vi "Dashboard Main.vi"() -> ()   [LabVIEW 2016]
uses:
  <vilib>/event_ctls.llb/eventvkey.ctl
  <vilib>/Rock Robotics/WPI/Dashboard/WPI_DashboardLogging Global.vi
  <vilib>/Utility/config.llb/Write Key (String).vi
  <vilib>/Utility/config.llb/Write Key (I32).vi
  <vilib>/Utility/config.llb/NI_LVConfig.lvlib
panel:
  out "Camera IP":string
  in  "TCP":refnum<k5>
  in  "Rec Mode":enum32{"Stop", "Record", "Playback"}(radio)
  in  "Vision":u16(ring) items=["Camera Off", "USB Camera SW", "USB Camera HW", "IP Camera"]
  out "Image Message":string="Timeout in Camera Communications"
  in  "Dashboard Tab":T1(tab)
  out "Feeder":bool
  out "GearPickupDown":bool caption="Gear Down"
  out "TargetLocked":bool caption="Locked"
  out "AutoTarget":bool caption="Target\nTarget"
  out "GearPickupMotor":bool caption="Gear Pickup"
  out "BallPickupMotor":bool caption="Ball Pickup"
  out "ShooterMotor":bool caption="Shooter"
  out "PTO":bool
  out "Neutral":bool
  out "High":bool caption="High Gear"
  out "Low":bool caption="Low Gear"
  in  "CompressorEnabled":bool caption="Compressor"
  out "Compressor":bool
  in  "AutoProgramSelect":u16(ring) items=["0 - No Auto Program", "1 - Drive to Line and Stop", "2 - Place Gear Center", "3 - Place Gear Start Left", "4 - Place Gear Start Right", "5 - Place Gear Vision Start Left", "6 - Place Gear Vision Start Right", "7 - Test Backwards Driving"]
  out "Low Battery":bool
  out "FMS":bool
  out "Teleop Mode":bool
  out "Auto Mode":bool
  out "Disabled":bool
  in  "Program":string
  in  "Camera Settings Old":T2={"Frame Rate"=30, "Compression"=30, "Size"=1, "Boolean"=FALSE} {"Frame Rate" scale=1.0..30.0; "Size" items=["640x480", "320x240", "160x120"]}
  out "Mode":T3(ring)=enum."Auto Disabled"
  in  "DB Camera Config":bool
  out "fps":dbl format="%#.1g"
  out "Mbps":dbl format="%#.1g"
  out "Mbps 2":bool
  in  "PIDEnabled":bool caption="PID Enabled"
  in  "LCD_Line_10":string caption="DB/String 0"
  in  "LCD_Line_9":string caption="DB/String 0"
  in  "LCD_Line_8":string caption="DB/String 0"
  in  "LCD_Line_7":string caption="DB/String 0"
  in  "LCD_Line_6":string caption="DB/String 0"
  in  "LCD_Line_5":string caption="DB/String 0"
  in  "LCD_Line_4":string caption="DB/String 0"
  in  "LCD_Line_3":string caption="DB/String 0"
  in  "LCD_Line_2":string caption="DB/String 0"
  in  "LCD_Line_1":string caption="DB/String 0"
  in  "PValue":dbl caption="P"
  in  "IValue":dbl caption="I"
  in  "DValue":dbl caption="D"
  in  "LowSetting":dbl caption="Low"
  in  "HighSetting":dbl caption="High"
  in  "DB/String 9":string
  in  "DB/String 8":string
  in  "DB/String 7":string
  in  "DB/String 6":string
  in  "DB/String 5":string
  in  "DB/String 4":string
  in  "DB/String 3":string
  in  "DB/String 2":string
  in  "DB/String 1":string
  in  "DB/String 0":string
  in  "DB/Slider 0":dbl(slide) scale=0.0..5.0
  in  "DB/Slider 1":dbl(slide) scale=0.0..5.0
  in  "DB/Slider 2":dbl(slide) scale=0.0..5.0
  in  "DB/Slider 3":dbl(slide) scale=0.0..5.0
  out "DB/LED 3":bool
  out "DB/LED 2":bool
  out "DB/LED 1":bool
  out "DB/LED 0":bool
  in  "DB/Button 3":bool
  in  "DB/Button 2":bool
  in  "DB/Button 1":bool
  in  "DB/Button 0":bool caption="New Name"
  in  "Test Slider":dbl(slide) scale=0.0..100.0 scale format="%#_3g"
  in  "On/Off":bool caption="Solenoid"
  in  "Test Name":u16(ring) items=["Select the test to run...", "Example Test", "-------------------------------", "List of tests is built in robot code.", "Replace with your own automated tests."]
  in  "Test Tree":string(tree)
  in  "Motor":cluster{"Value":dbl, "Enable":bool} {"Value" scale=-1.0..1.0 scale format="%#_3g"}
  out "Progress":T4 {"Test Progress" scale=0.0..100.0}
  in  "Rev/Fwd":cluster{"Forward":bool, "Reverse":bool}
  in  "Test Ring":u16(ring) items=["Monochrome", "Color"]
  in  "Listbox":i32(listbox)
  out "Tree":string(tree)
  out "Camera Image":T5(plugin-control)
  out "Boolean":bool
  # "Program:"
  # "Dashboard: 2017-04"
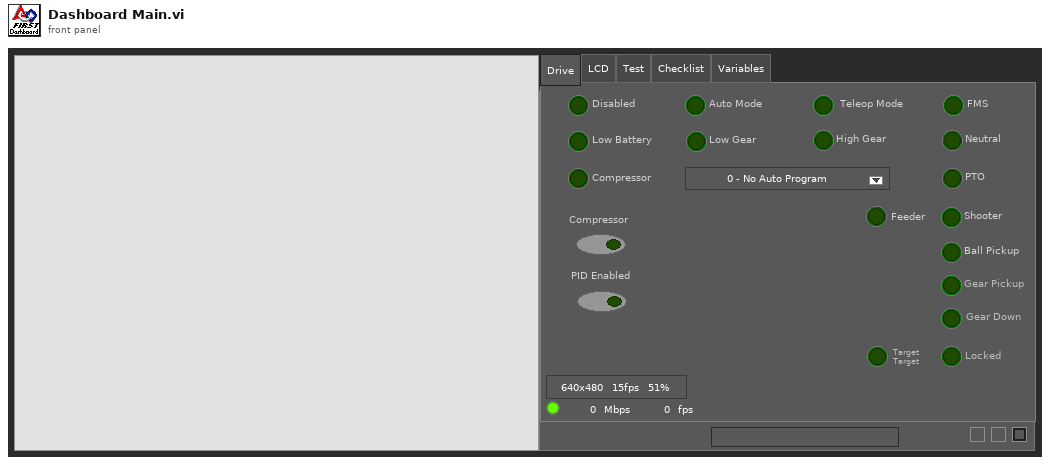
[diagram p1: front panel]
types:
  T1 = enum32{"Drive", "LCD", "Basic", "Test", "Checklist", "Variables"}
  T2 = cluster{"Frame Rate":i32, "Compression":i32, "Size":u16, "Boolean":bool}
  T3 = enum8{"Tele-Op Disabled", "Tele-Op Enabled", "Auto Disabled", "Auto Enabled", "Test Disabled", "Test Enabled", "Disconnected", "No Code", "E-Stop"}
  T4 = cluster{"Test Progress":u8, "Test Progress Text":string}
  T5 = typedef "IMAQ Image.ctl" = refnum<image>
  T6 = enum32{"Drive", "Basic", "Custom", "Test", "Checklist", "Variables"}
  T7 = typedef "Image Type" = u32
  T8 = cluster{"Camera Image":refnum<vi>, "Dashboard Tab":refnum<vi>, "Boolean":refnum<vi>, "Vision":refnum<vi>, "Rec Mode":refnum<vi>, "Test Slider":refnum<vi>, "On/Off ":refnum<vi>, "Test Ring":refnum<vi>, "Rev/Fwd":refnum<vi>, "Test Name":refnum<vi>, "Motor":refnum<vi>, "Progress":refnum<vi>, "CheckList":refnum<vi>, "Tree":refnum<vi>, "Test Tree":refnum<vi>}
  T9 = cluster{"Error Strings":string, "Disable Counts":cluster{u16, u16}, "Rail Faults":cluster{u16, u16, u16}, "Robot IP":string, "DB Mode":u8, "Event Info":cluster{"Name":string, "Type":u8, "Number":u16, "Replay":u8}}
  T10 = cluster{"Storage":cluster{"Disk Free":u64, "RAM Block":u32, "RAM free":u32}, "CPU Utilization":cluster{"CPU % ISR":sgl, "CPU % Time Crit":sgl, "CPU % Timed Str":sgl, "CPU % High":sgl, "CPU % Above":sgl, "CPU % Normal":sgl, "CPU % Low":sgl}, "CAN":cluster{"% Bus Utilization":sgl, "Bus Off Cnt":u32, "TX_FIFO Full Cnt":u32, "Receive Error Cnt":u8, "Transmit Error Cnt":u8}, "HID":cluster{"HID Outputs":u32, "Rumble Low":u16, "Rumble High":u16}[]}
  T11 = cluster{"Status bits":cluster{"Test Mode":bool, "Autonomous":bool, "Enabled":bool, "Code Start":bool, "Brownout":bool, "Reserved 2":bool, "Reserved 3":bool, "E-Stop":bool}, "Code Trace":cluster{"Disabled":bool, "TeleOp":bool, "Auto":bool, "Test":bool}, "Controller Type":enum16{"unknown", "cRIO", "roboRio"}, "Code?":enum16{"unknown", "noCode", "code"}, "Battery V":dbl}
  T12 = cluster{"Control Bits":cluster{"TestMode":bool, "Autonomous":bool, "Enabled":bool, "FMS Present":bool, bool, bool, bool, "E-Stop":bool}, "Team Station ":u8, "Countdown":sgl, "Joystick Values":cluster{"Axes":dbl[], "Buttons":bool[], "POVs":i16[]}[]}
  T13 = cluster{"value":i32, "value":i32, "index":i32, "Boolean":bool}
  T14 = typedef "NI_LVConfig.lvlib/Config Data RefNum.ctl" = refnum<k1>
  T15 = cluster{"Operation":enum16{"Update", "Clear"}, "Color Box":u32}[]
  T16 = typedef "eventvkey.ctl" = enum16{"ASCII", "Enter", "Return", "Shift", "Ctrl", "Alt", "Cmd", "Opt", "Caps", "NumLock", "Clear", "Break", "Up", "Down", "Left", "Right", "Insert", "Delete", "Home", "End", "PageUp", "PageDown", "Escape", "Help", "Pause", "ScrollLock", "F1", "F2", "F3", "F4", "F5", "F6", "F7", "F8", "F9", "F10", "F11", "F12", "F13", "F14", "F15", "F16", "F17", "F18", "F19", "F20", "F21", "F22", "F23", "F24", "Play", "VolumeUp", "VolumeDown", "Mute", "Two Byte Char"}
  T17 = cluster{"Image Size":bool, "Image Type":bool, "Pixel Value":bool, "ROI Information":bool, "Zoom Factor":bool}
  T18 = enum8{"Enabled", "Disabled", "Disabled and Grayed Out"}
  T19 = cluster{"Operation":enum16{"Update", "Clear"}, "Color Box":u32}
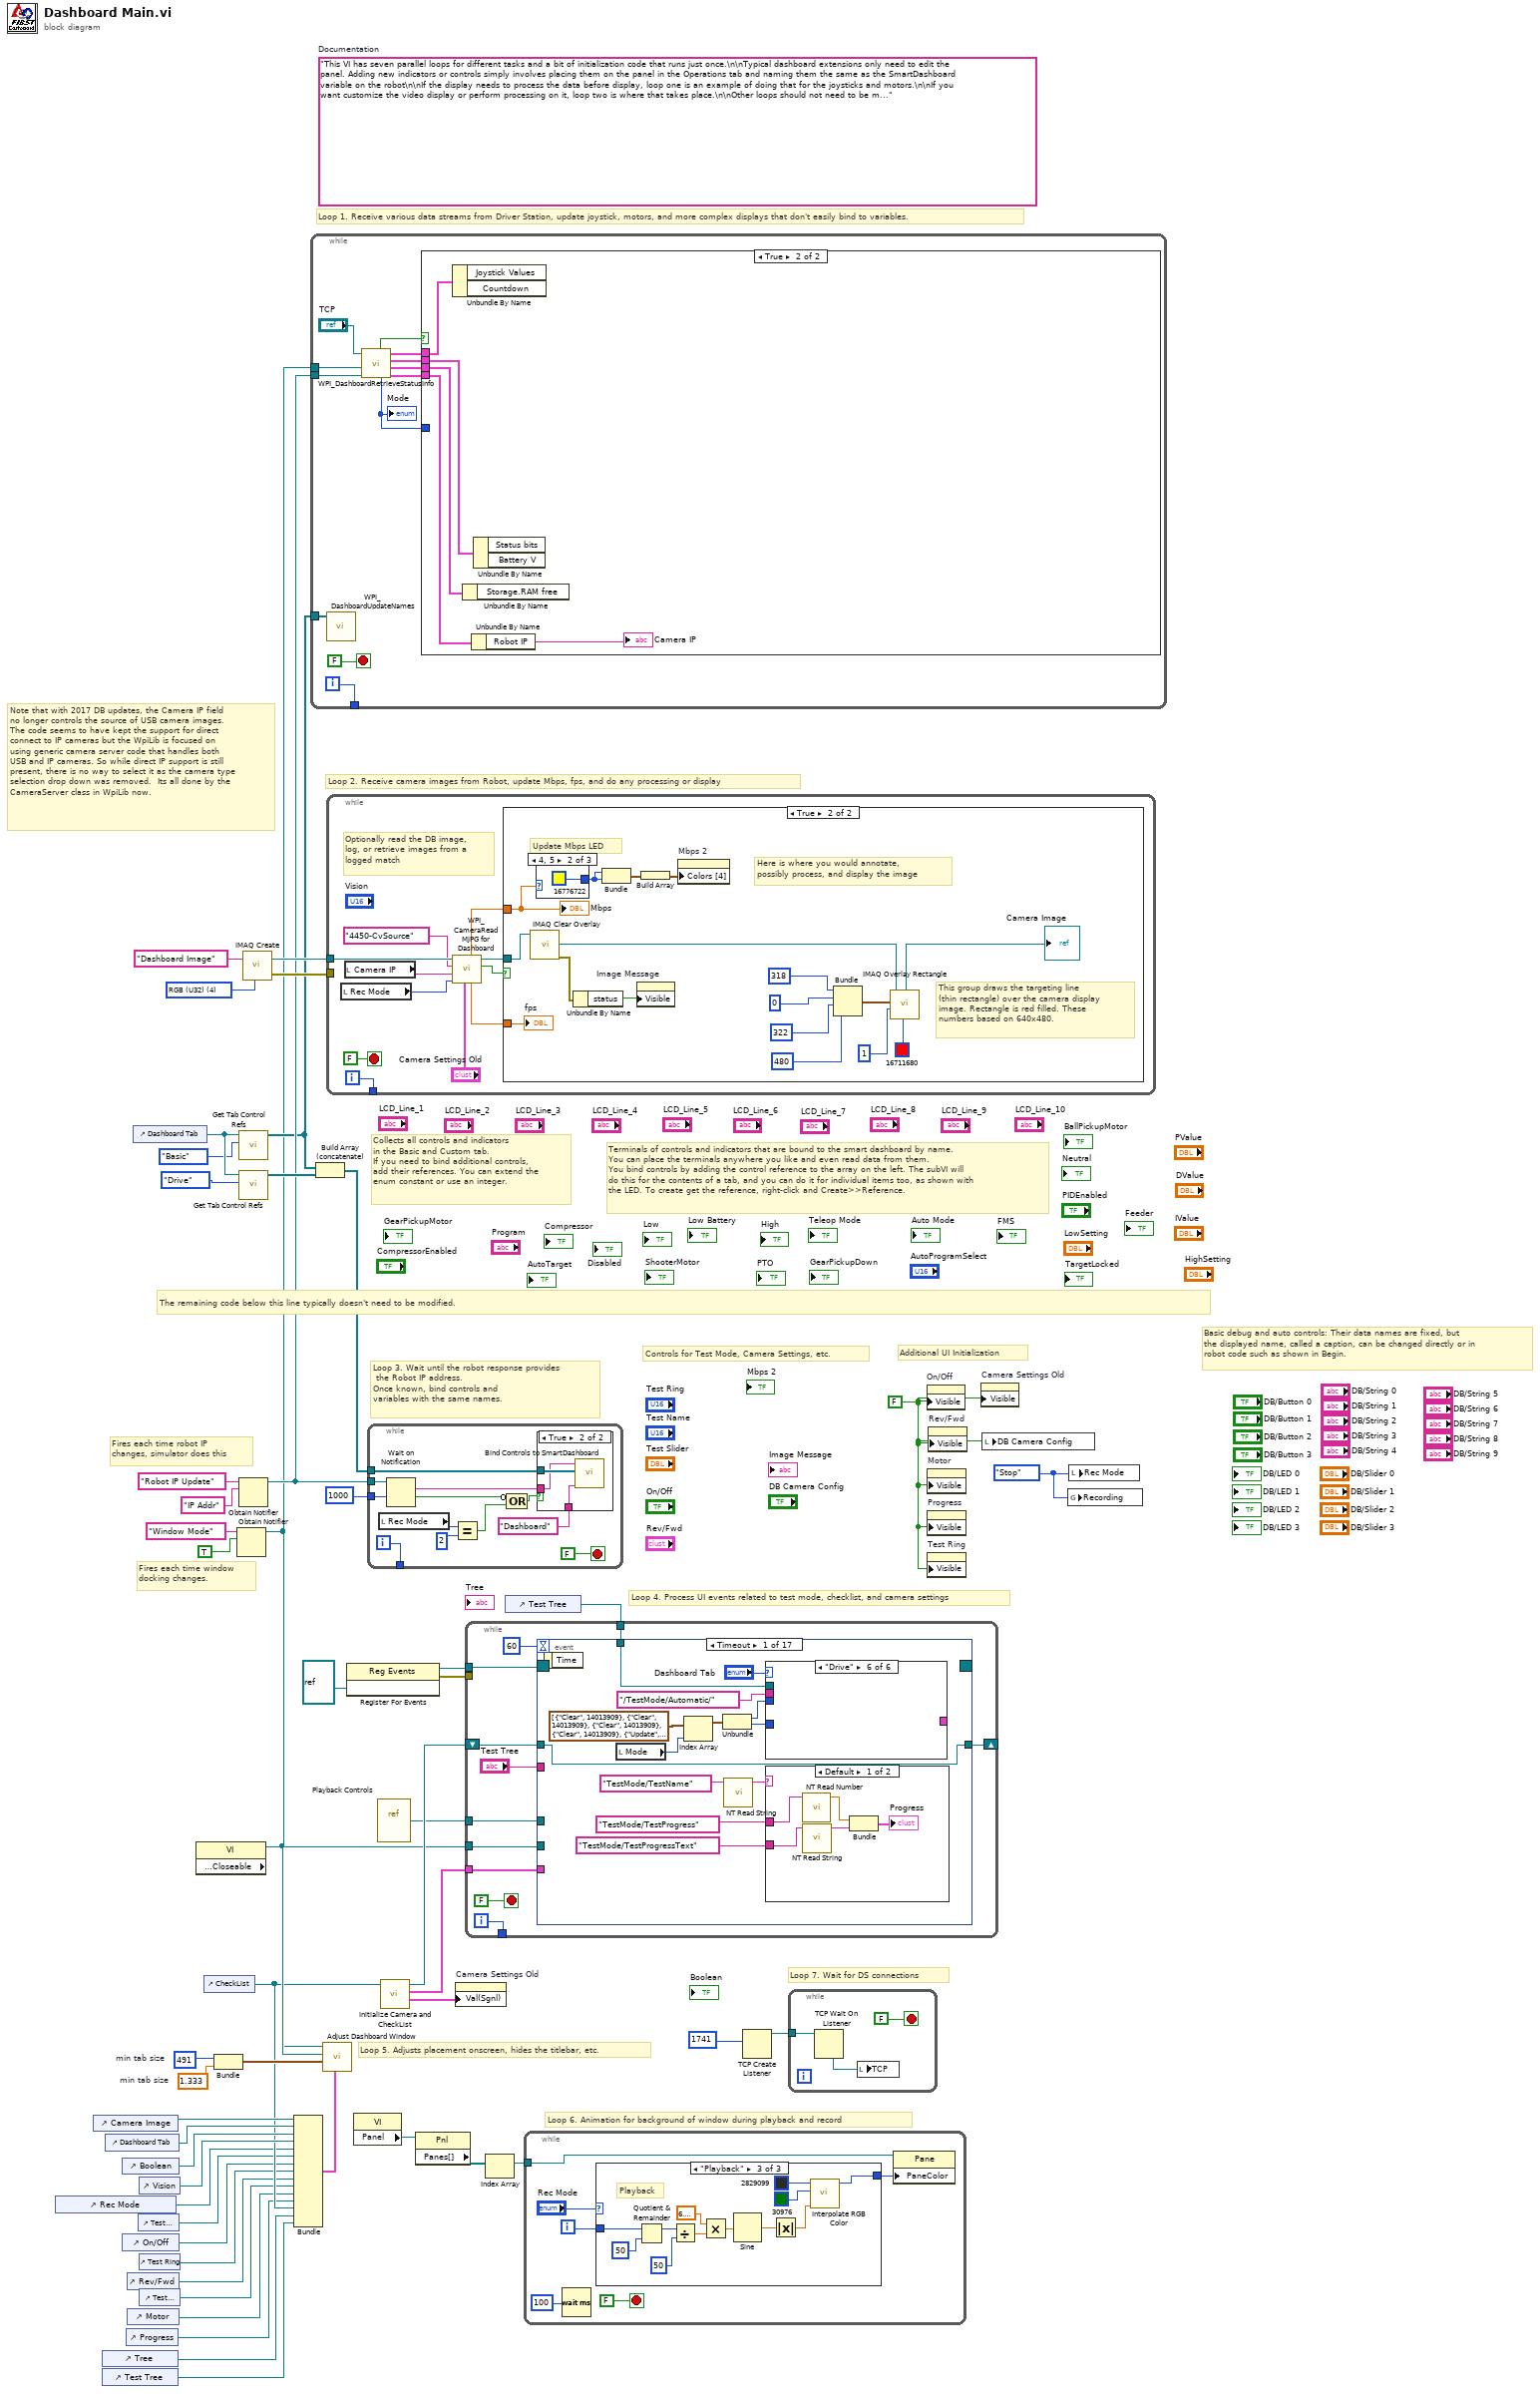
[diagram p0: block diagram]
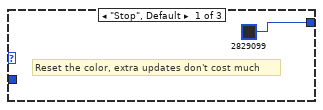
[diagram p3: hidden frame]
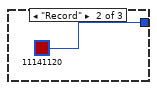
[diagram p4: hidden frame]
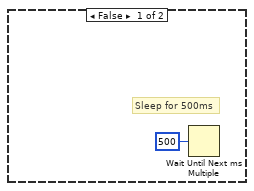
[diagram p6: hidden frame]
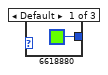
[diagram p7: hidden frame]
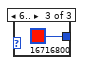
[diagram p8: hidden frame]
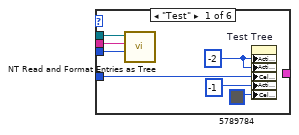
[diagram p9: hidden frame]
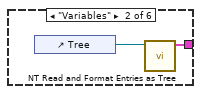
[diagram p10: hidden frame]
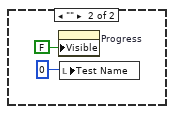
[diagram p14: hidden frame]
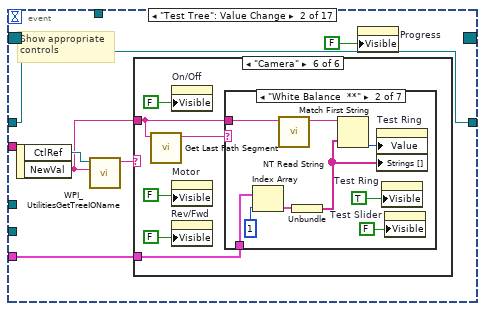
[diagram p15: hidden frame]
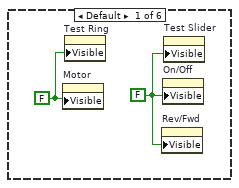
[diagram p16: hidden frame]
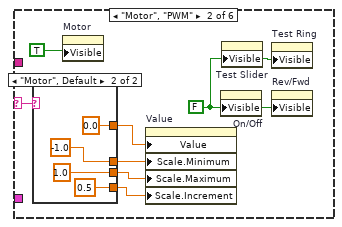
[diagram p17: hidden frame]
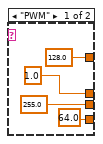
[diagram p18: hidden frame]
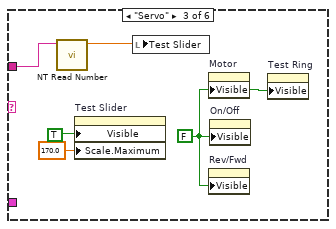
[diagram p19: hidden frame]
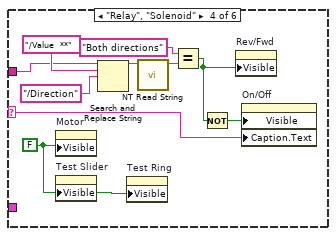
[diagram p20: hidden frame]
diagram:
  w24 = 491  # min tab size
  w23 = 1.333  # min tab size
  w32 = enum32{"Stop", "Record", "Playback"}."Stop" ("Rec Mode")
  w6 = FALSE ("Visible")
  (unwired) "This VI has seven parallel loops for different tasks and a bit of initialization code that runs just once.\n\nTypical dashboard extensions only need to edit the panel. Adding new indicators or controls simply involves placing them on the panel in the Operations tab and naming them the same as the SmartDashboard variable on the robot\n\nIf the display needs to process the data before display, loop one is an example of doing that for the joysticks and motors.\n\nIf you want customize the video display or perform processing on it, loop two is where that takes place.\n\nOther loops should not need to be modified. They are pretty standard, and document the task they perform."  # Documentation
  w52 = T7 4 items=["Grayscale (U8)", "Grayscale (I16)", "Grayscale (SGL)", "Complex (CSG)", "RGB (U32)", "HSL (U32)", "RGB (U64)"] ("Image Type")
  # "Note that with 2017 DB updates, the Camera IP field\nno longer controls the source of USB camera images.\nThe code seems to have kept the support for direct\nconnect to IP cameras but the WpiLib is focused on\nusing generic camera server code that handles both\nUSB and IP cameras. So while direct IP support is still\npresent, there is no way to select it as the camera type\nselection drop down was removed.  Its all done by the\nCameraServer class in WpiLib now."
  # "Loop 7. Wait for DS connections"
  # "Basic debug and auto controls: Their data names are fixed, but\nthe displayed name, called a caption, can be changed directly or in\nrobot code such as shown in Begin."
  # "Controls for Test Mode, Camera Settings, etc."
  # "Additional UI Initialization"
  # "Loop 6. Animation for background of window during playback and record"
  # "Fires each time robot IP\nchanges, simulator does this"
  # "Fires each time window\ndocking changes."
  # "Collects all controls and indicators\nin the Basic and Custom tab.\nIf you need to bind additional controls,\nadd their references. You can extend the\nenum constant or use an integer."
  # "The remaining code below this line typically doesn't need to be modified."
  # "Loop 4. Process UI events related to test mode, checklist, and camera settings"
  # "Terminals of controls and indicators that are bound to the smart dashboard by name.\nYou can place the terminals anywhere you like and even read data from them.\nYou bind controls by adding the control reference to the array on the left. The subVI will\ndo this for the contents of a tab, and you can do it for individual items too, as shown with\nthe LED. To create get the reference, right-click and Create>>Reference."
  # "Loop 3. Wait until the robot response provides\n the Robot IP address.\nOnce known, bind controls and\nvariables with the same names."
  # "Loop 5. Adjusts placement onscreen, hides the titlebar, etc."
  # "Loop 1. Receive various data streams from Driver Station, update joystick, motors, and more complex displays that don't easily bind to variables."
  # "Loop 2. Receive camera images from Robot, update Mbps, fps, and do any processing or display"
  n1 = control-ref of="Rec Mode"() -> (w12:refnum<vi>)
  n2 = control-ref of="Camera Image"() -> (w27:refnum<vi>)
  n3 = control-ref of="Tree"() -> (w16:refnum<vi>)
  n4 = control-ref of="Test Tree"() -> (w15:refnum<vi>)
  n5 = control-ref of="Dashboard Tab"() -> (w26:refnum<vi>)
  n6 = control-ref of="Boolean"() -> (w21:refnum<vi>)
  n7 = control-ref of="On/Off"() -> (w10:refnum<vi>)
  n8 = control-ref of="Progress"() -> (w7:refnum<vi>)
  n9 = control-ref of="Rev/Fwd"() -> (w8:refnum<vi>)
  n10 = control-ref of="Motor"() -> (w13:refnum<vi>)
  n11 = control-ref of="Dashboard Tab"() -> (w30:refnum<vi>)
  n12 = control-ref of="Test Slider"() -> (w11:refnum<vi>)
  n13 = control-ref of="Vision"() -> (w25:refnum<vi>)
  n14 = control-ref of="Test Ring"() -> (w9:refnum<vi>)
  n15 = control-ref of="Test Name"() -> (w14:refnum<vi>)
  n16 = property class="VI" props=["Front Panel.Closeable"]() -> (reference out=w31:refnum<vi>)  [unwired: 2 in, 2 out]
  n17 = control-ref of="CheckList"() -> (w17:refnum<vi>)
  n18 = Bundle("min tab size"=w24, "min tab size"=w23) -> (w22:cluster{"min tab size":i32, "min tab size":dbl})  [unwired: 1 in]
  n19 = Obtain Notifier(name (unnamed)="Window Mode", notification data type=TRUE) -> (notifier out=w3:refnum<notifier>)  [unwired: 2 in, 2 out]
  n20 = call <vilib>:"Get Tab Control Refs.vi"("Page Index"=T6."Basic" ("Dashboard Tab"), "TabControl in"=w30) -> ("ControlsOnPage"=w4:refnum<vi>[])  [unwired: 9 in]
  n21 = call <vilib>:"Get Tab Control Refs.vi"("Page Index"=T6."Drive" ("Dashboard Tab"), "TabControl in"=w30) -> ("ControlsOnPage"=w29:refnum<vi>[])  [unwired: 9 in]
  n22 = Obtain Notifier(name (unnamed)="Robot IP Update", notification data type="IP Addr" ("name (unnamed)")) -> (notifier out=w5:refnum<notifier>)  [unwired: 2 in, 2 out]
  n23 = call "IMAQ Create"("Image Name"="Dashboard Image", "Image Type"=w52) -> ("New Image"=w50:T5, "error out"=w49:errorcluster)  [unwired: 2 in, 1 out]
  n24 = Bundle("Camera Image"=w27, "Dashboard Tab"=w26, "Boolean"=w21, "Vision"=w25, "Rec Mode"=w12, "Test Slider"=w11, "On/Off"=w10, "Test Ring"=w9, "Rev/Fwd"=w8, "Test Name"=w14, "Motor"=w13, "Progress"=w7, "CheckList"=w17, "Tree"=w16, "Test Tree"=w15) -> (w18:T8)  [unwired: 1 in]
  n25 = while {
    tunnel: [w63] -> _
    tunnel: w5 -> [w57]
    tunnel: w4 -> [w56]
    tunnel: w3 -> [w53]
    i -> [w63]
    stop <- FALSE stop-if-true
    n26 = call <vilib>:"WPI_DashboardUpdateNames.vi"("Controls on Tab"=w56) -> ()  [unwired: 11 in]
    n27 = call <vilib>:"WPI_DashboardRetrieveStatusInfo.vi"("Binding Refnum"=w57, "Window Mode Notifier"=w53, "TCP Cnx"="TCP") -> ("Power and Errors"=w58:T9, "Robot Metrics"=w61:T10, "Status Info"=w62:T11, "Control Info"=w59:T12, "Robot Mode"=w55:T3, "Process?"=w60:bool)  [unwired: 3 in]
    "Mode" <- w55
    n28 = case shown="True" w60 {
      tunnel: w62 -> [_ w69]
      tunnel: w61 -> [_ w68]
      tunnel: w59 -> [_ w67]
      tunnel: w58 -> [_ w66]
      tunnel: w55 -> [_ _]
      frame False {
      }
      frame True {
        n29 = Unbundle By Name(w67) -> ()  [unwired: 2 out]
        n30 = Unbundle By Name(w68) -> ()  [unwired: 1 out]
        n31 = Unbundle By Name(w66) -> ("Robot IP"=→"Camera IP":string)
        n32 = Unbundle By Name(w69) -> ()  [unwired: 2 out]
      }
    }
  }
  n33 = Build Array (concatenate)(w4, w29) -> (w28:refnum<vi>[])
  n34 = call "Adjust Dashboard Window.vi"("Sizing Refnums"=w18, "Size Constraints"=w22, "VI"=w31, "Notifier in"=w3) -> ()  [unwired: 8 in]
  n35 = while {
    tunnel: w50 -> [w78]
    tunnel: w49 -> [_]
    tunnel: [w79] -> _
    i -> [w79]
    stop <- FALSE stop-if-true
    # "Optionally read the DB image,\nlog, or retrieve images from a\nlogged match"
    n36 = local read "Rec Mode"() -> (w73:enum32{"Stop", "Record", "Playback"})
    n37 = local read "Camera IP"() -> (w72:string)
    n38 = call <vilib>:"WPI_CameraRead MJPG for Dashboard.vi"("Camera Settings"="Camera Settings Old", "Rec Mode"=w73, "Robot IP"=w72, "Camera Name"="4450-CvSource", "Refnum in"=w78) -> ("Active"=w76:bool, "Refnum out"=w77:T5, "FPS"=w75:dbl, "Bandwidth (Mbps)"=w74:dbl)  [unwired: 3 in]
    n39 = case shown="True" w76 {
      tunnel: w77 -> [_ w93]
      tunnel: w74 -> [_ w92]
      tunnel: w75 -> [_ w91]
      frame False {
        # "Sleep for 500ms"
        n40 = Wait Until Next ms Multiple(millisecond multiple=u32 500) -> ()  [unwired: 1 out]
      }
      frame True {
        # "This group draws the targeting line\n(thin rectangle) over the camera display\nimage. Rectangle is red filled. These\nnumbers based on 640x480."
        # "Here is where you would annotate,\npossibly process, and display the image"
        # "Update Mbps LED"
        n41 = call "IMAQ Clear Overlay"("Image"=w93) -> ("error out"=w97:errorcluster, "Image Out"=w83:T5)  [unwired: 2 in, 7 out]
        n42 = case shown="4, 5" w92 {
          tunnel: [u32 6618880 ("Color Box") u32 16776722 ("Color Box") u32 16716800 ("Color Box")] -> w94
          frame Default {
          }
          frame 4, 5 {
          }
          frame 6.. {
          }
        }
        n43 = Unbundle By Name(w97) -> ("status"=w98:bool)
        n44 = Bundle("Color Box"=w94, "Color Box"=w94) -> (w96:cluster{"Color Box":u32, "Color Box":u32})  [unwired: 1 out]
        n45 = property on="Image Message" class="Str"("Visible"=w98) -> ()  [unwired: 2 in, 2 out]
        n46 = Build Array(w96) -> (w95:cluster{"Color Box":u32, "Color Box":u32}[])
        n47 = property on="Mbps 2" class="Bool (strict)"("Colors [4]"=w95) -> ()  [unwired: 2 in, 2 out]
        n48 = Bundle(318, 0, 322, 480) -> (w89:cluster{i32, i32, i32, i32})  [unwired: 1 out]
        n49 = call "IMAQ Overlay Rectangle"("Color"=u32 16711680, "Drawing Mode (Frame)"=1, "Rectangle"=w89, "Image"=w83) -> ("Image Out"=→"Camera Image":T5)  [unwired: 6 in, 1 out]
        "Mbps" <- w92
        "fps" <- w91
      }
    }
  }
  n50 = register-events(refnum<vi> refnum) -> (reference out=w36:refnum<event-registration>, error out=w35:errorcluster)  [unwired: 2 in]
  n51 = property class="VI"() -> ("Panel"=w39:refnum<vi>)  [unwired: 2 in, 2 out]
  n52 = while {
    tunnel: w28 -> [w113]
    tunnel: w5 -> [w111]
    tunnel: [w109] -> _
    tunnel: u32 1000 ("milliseconds to wait") -> [w108]
    i -> [w109]
    stop <- FALSE stop-if-true
    n53 = local read "Rec Mode"() -> (w104:enum32{"Stop", "Record", "Playback"})
    n54 = Wait on Notification(notifier=w111, timeout in ms (-1)=w108) -> (notification=w110:string, timed out?=w106:bool)  [unwired: 2 in, 2 out]
    n55 = Equal?(x=w104, y=u16 2 ("Rec Mode")) -> (x = y?=w105:bool)
    n56 = Compound Arithmetic op=OR(invert w106, w105) -> (w107:bool)
    n57 = case shown="True" w107 {
      tunnel: w113 -> [_ w116]
      tunnel: w110 -> [_ w115]
      tunnel: "Dashboard" -> [_ w114]
      frame False {
      }
      frame True {
        n58 = call <vilib>:"Bind Controls to SmartDashboard.vi"("Client Name"=w114, "Bound Control Refs"=w116, "Server IP Address"=w115) -> ()  [unwired: 9 in]
      }
    }
  }
  n59 = vi-ref "Playback Controls.vi"() -> (w37:refnum<vi>)
  n60 = call "Initialize Camera and CheckList.vi"("ListBox in"=w17) -> ("Cluster"=w43:T13, "Array"=w44:cluster{string[]}[], "File Refnum"=w42:T14)  [unwired: 7 in, 1 out]
  n61 = property class="Pnl"(reference=w39) -> ("Panes[]"=w40:refnum<vi>[])  [unwired: 1 in, 2 out]
  n62 = property on="Camera Settings Old" class="Clust (strict)"("Val(Sgnl)"=w43) -> ()  [unwired: 2 in, 2 out]
  n63 = Index Array(array=w40) -> (element=w38:refnum<vi>)  [unwired: 1 in]
  n64 = control-ref of="Test Tree"() -> (w41:refnum<vi>)
  n65 = while {
    tunnel: w44 -> [w124]
    shift-right: [w123] -> _
    shift-left: w42 -> [w122]
    tunnel: [w121] -> _
    tunnel: w41 -> [w120]
    tunnel: w37 -> [w119]
    tunnel: w36 -> [w118]
    tunnel: w35 -> [_]
    tunnel: w31 -> [w117]
    i -> [w121]
    stop <- FALSE stop-if-true
    n66 = event shown="[0] Timeout" {
      selector: w118 -> [_ _ _ _ _ _ _ _ _ _ _ _ _ _ _ _ _]
      dyn-events: [_ _ _ _ _ _ _ _ _ _ _ _ _ w362 _ _ _] -> _
      timeout: u32 60 ("milliseconds to wait") -> [_ _ _ _ _ _ _ _ _ _ _ _ _ _ _ _ _]
      tunnel: w120 -> [w136 _ _ _ _ _ _ _ _ _ _ _ _ _ _ _ _]
      tunnel: "Test Tree" -> [_ _ _ _ _ _ _ _ w331 w339 w341 w345 w353 _ _ _ _]
      tunnel: w124 -> [_ w158 _ _ _ _ w295 w325 _ _ _ _ _ _ _ _ _]
      tunnel: [w132 w157 w256 w261 w269 w281 w294 w318 w330 w337 w340 w344 w352 w364 w378 w379 w389] -> w123
      tunnel: w122 -> [w132 w157 w256 w261 w269 w281 w293 w318 w330 w337 w340 w344 w352 w364 w378 w379 w389]
      tunnel: w119 -> [_ _ _ _ _ _ _ _ _ _ _ _ _ w365 _ w382 _]
      tunnel: w117 -> [_ _ _ _ _ _ _ _ _ _ _ _ _ w360 _ _ _]
      event Timeout {
        n67 = event-data() -> ()  [unwired: 1 in, 1 out]
        n68 = local read "Mode"() -> (w135:T3)
        n69 = Index Array(array=T15 [{"Operation"=enum."Clear", "Color Box"=14013909}, {"Operation"=enum."Clear", "Color Box"=14013909}, {"Operation"=enum."Clear", "Color Box"=14013909}, {"Operation"=enum."Clear", "Color Box"=14013909}, {"Operation"=enum."Update", "Color Box"=14013909}, {"Operation"=enum."Update", "Color Box"=16777215}, {"Operation"=enum."Clear", "Color Box"=14013909}, {"Operation"=enum."Clear", "Color Box"=14013909}, {"Operation"=enum."Clear", "Color Box"=14013909}], index=w135) -> (element=w130:T19)
        n70 = Unbundle(w130) -> ("Operation"=w129:enum16{"Update", "Clear"}, "Color Box"=w128:u32)
        n71 = call <vilib>:"NT Read String.vi"("Name"="TestMode/TestName") -> ("String"=w139:string)  [unwired: 9 in, 1 out]
        n72 = case shown="\"Drive\"" "Dashboard Tab" {
          tunnel: w136 -> [w147 _ _ _ _ _]
          tunnel: "/TestMode/Automatic/" ("Name Pattern") -> [w146 _ _ _ _ _]
          tunnel: w129 -> [w145 _ _ _ _ _]
          tunnel: [_ w149 _ _ _ _] -> _
          tunnel: w128 -> [w141 _ _ _ _ _]
          frame "Test" {
            w144 = -2 ("Active Item:Row Number")
            n73 = call <vilib>:"NT Read and Format Entries as Tree.vi"("Operation"=w145, "Name Pattern"=w146, "Tree Refnum"=w147) -> ()  [unwired: 7 in, 2 out]
            n74 = property on="Test Tree" class="Tree (strict)"("Active Item Row Number"=w144, "ActiveColNum"=w144, "CellBG"=w141, "Active Item Row Number"=-1 ("Active Item:Row Number"), "CellBG"=u32 5789784 ("Color Box")) -> ()  [unwired: 2 in, 2 out]
          }
          frame "Variables" {
            n75 = control-ref of="Tree"() -> (w148:refnum<vi>)
            n76 = call <vilib>:"NT Read and Format Entries as Tree.vi"("Tree Refnum"=w148) -> ("Formatted Strings"=w149:cluster{"Name":string, "Value":string}[])  [unwired: 9 in, 1 out]
          }
          frame "Checklist" {
          }
          frame "Basic" {
          }
          frame "LCD" {
          }
          frame "Drive" {
          }
        }
        n77 = case shown="Default" w139 {
          tunnel: "TestMode/TestProgress" ("Name") -> [w151 _]
          tunnel: "TestMode/TestProgressText" ("Name") -> [w150 _]
          frame Default {
            n78 = call <vilib>:"NT Read Number.vi"("Name"=w151) -> ("Numeric"=w152:dbl)  [unwired: 9 in, 1 out]
            n79 = call <vilib>:"NT Read String.vi"("Name"=w150) -> ("String"=w153:string)  [unwired: 9 in, 1 out]
            n80 = Bundle("Numeric"=w152, "String"=w153) -> (→"Progress":cluster{"Numeric":dbl, "String":string})  [unwired: 1 in]
          }
          frame "" {
            n81 = property on="Progress" class="Clust (strict)"("Visible"=FALSE) -> ()  [unwired: 2 in, 2 out]
            n82 = local write "Test Name"(u16 0) -> ()
          }
        }
      }
      event "Test Tree": Value Change {
        # "Show appropriate\ncontrols"
        n83 = event-data() -> ("CtlRef"=w161:refnum<vi>, "NewVal"=w159:string)  [unwired: 1 in]
        n84 = call <vilib>:"WPI_UtilitiesGetTreeIOName.vi"("NewVal"=w159, "TreeControl in"=w161) -> ("I/O Name"=w162:string)  [unwired: 9 in]
        n85 = case shown="\"Camera\"" w162 {
          selector: w162 -> [_ w169 _ w187 w196 _]
          tunnel: w159 -> [_ _ w184 w186 _ w203]
          tunnel: w158 -> [_ _ _ _ _ w202]
          frame Default {
            w164 = FALSE ("Visible")
            w163 = FALSE ("Visible")
            n86 = property on="Motor" class="Clust (strict)"("Visible"=w163) -> ()  [unwired: 2 in, 2 out]
            n87 = property on="Test Ring" class="Ring (strict)"("Visible"=w163) -> ()  [unwired: 2 in, 2 out]
            n88 = property on="Rev/Fwd" class="Clust (strict)"("Visible"=w164) -> ()  [unwired: 2 in, 2 out]
            n89 = property on="On/Off" class="Bool (strict)"("Visible"=w164) -> ()  [unwired: 2 in, 2 out]
            n90 = property on="Test Slider" class="Slide (strict)"("Visible"=w164) -> ()  [unwired: 2 in, 2 out]
          }
          frame "Motor", "PWM" {
            w170 = FALSE ("Visible")
            n91 = case shown="\"Motor\", Default" w169 {
              tunnel: [1.0 ("Value") -1.0 ("Value")] -> w168
              tunnel: [255.0 ("Value") 1.0 ("Value")] -> w167
              tunnel: [128.0 ("Value") 0.0 ("Value")] -> w166
              tunnel: [64.0 ("Value") 0.5 ("Value")] -> w165
              frame "PWM" {
              }
              frame "Motor", Default {
              }
            }
            n92 = property on="Motor" class="Clust (strict)"("Visible"=TRUE) -> ()  [unwired: 2 in, 2 out]
            n93 = property on="Value" class="Slide (strict)"("Value"=w166, "Scale.Minimum"=w168, "Scale.Maximum"=w167, "Scale.Increment"=w165) -> ()  [unwired: 2 in, 2 out]
            n94 = property on="On/Off" class="Bool (strict)"("Visible"=w170) -> ()  [unwired: 2 in, 2 out]
            n95 = property on="Test Slider" class="Slide (strict)"("Visible"=w170) -> ()  [unwired: 2 in, 2 out]
            n96 = property on="Test Ring" class="Ring (strict)"("Visible"=w170) -> ()  [unwired: 2 in, 2 out]
            n97 = property on="Rev/Fwd" class="Clust (strict)"("Visible"=w170) -> ()  [unwired: 2 in, 2 out]
          }
          frame "Servo" {
            w182 = FALSE ("Visible")
            n98 = call <vilib>:"NT Read Number.vi"("Name"=w184) -> ("Numeric"=w183:dbl)  [unwired: 9 in, 1 out]
            n99 = property on="Test Slider" class="Slide (strict)"("Visible"=TRUE, "Scale.Maximum"=170.0 ("Scale.Range:Maximum")) -> ()  [unwired: 2 in, 2 out]
            n100 = local write "Test Slider"(w183) -> ()
            n101 = property on="Motor" class="Clust (strict)"("Visible"=w182) -> ()  [unwired: 2 in, 2 out]
            n102 = property on="Rev/Fwd" class="Clust (strict)"("Visible"=w182) -> ()  [unwired: 2 in, 2 out]
            n103 = property on="On/Off" class="Bool (strict)"("Visible"=w182) -> ()  [unwired: 2 in, 2 out]
            n104 = property on="Test Ring" class="Ring (strict)"("Visible"=w182) -> ()  [unwired: 2 in, 2 out]
          }
          frame "Relay", "Solenoid" {
            w185 = FALSE ("Visible")
            n105 = property on="Motor" class="Clust (strict)"("Visible"=w185) -> ()  [unwired: 2 in, 2 out]
            n106 = property on="Test Slider" class="Slide (strict)"("Visible"=w185) -> ()  [unwired: 2 in, 2 out]
            n107 = Search and Replace String(input string=w186, search string="/Value  **", replace string="/Direction") -> (result string=w192:string)  [unwired: 5 in, 3 out]
            n108 = property on="Test Ring" class="Ring (strict)"("Visible"=w185) -> ()  [unwired: 2 in, 2 out]
            n109 = call <vilib>:"NT Read String.vi"("Name"=w192) -> ("String"=w190:string)  [unwired: 9 in, 1 out]
            n110 = Equal?(x="Both directions", y=w190) -> (x = y?=w188:bool)
            n111 = Not(x=w188) -> (.not. x?=w189:bool)
            n112 = property on="Rev/Fwd" class="Clust (strict)"("Visible"=w188) -> ()  [unwired: 2 in, 2 out]
            n113 = property on="On/Off" class="Bool (strict)"("Visible"=w189, "Caption.Text"=w187) -> ()  [unwired: 2 in, 2 out]
          }
          frame "Compressor", "Digital Out" {
            w195 = FALSE ("Visible")
            # "Get direction and finish"
            n114 = property on="Motor" class="Clust (strict)"("Visible"=w195) -> ()  [unwired: 2 in, 2 out]
            n115 = property on="Test Slider" class="Slide (strict)"("Visible"=w195) -> ()  [unwired: 2 in, 2 out]
            n116 = property on="Test Ring" class="Ring (strict)"("Visible"=w195) -> ()  [unwired: 2 in, 2 out]
            n117 = property on="On/Off" class="Bool (strict)"("Visible"=TRUE, "Caption.Text"=w196) -> ()  [unwired: 2 in, 2 out]
            n118 = property on="Rev/Fwd" class="Clust (strict)"("Visible"=FALSE) -> ()  [unwired: 2 in, 2 out]
          }
          frame "Camera" {
            n119 = call <vilib>:"Get Last Path Segment.vi"("String in"=w203) -> ("String out"=w204:string)  [unwired: 10 in]
            n120 = property on="On/Off" class="Bool (strict)"("Visible"=FALSE) -> ()  [unwired: 2 in, 2 out]
            n121 = property on="Motor" class="Clust (strict)"("Visible"=FALSE) -> ()  [unwired: 2 in, 2 out]
            n122 = property on="Rev/Fwd" class="Clust (strict)"("Visible"=FALSE) -> ()  [unwired: 2 in, 2 out]
            n123 = case shown="\"White Balance  **\"" w204 {
              tunnel: w203 -> [w210 w219 w228 w237 w246 _ w252]
              tunnel: w202 -> [w208 w216 w225 w234 w243 _ _]
              frame "Size  **" {
                n124 = Index Array(array=w208) -> (element=w207:cluster{string[]})  [unwired: 1 in]
                n125 = call <vilib>:"NT Read String.vi"("Name"=w210) -> ("String"=w209:string)  [unwired: 9 in, 1 out]
                n126 = Unbundle(w207) -> (w205:string[])
                n127 = Match First String(2:w205, 3:w209) -> (0:w206:i32)  [unwired: 1 out]
                n128 = property on="Test Ring" class="Ring (strict)"("Value"=w206, "Strings []"=w205) -> ()  [unwired: 2 in, 2 out]
                n129 = property on="Test Ring" class="Ring (strict)"("Visible"=TRUE) -> ()  [unwired: 2 in, 2 out]
                n130 = property on="Test Slider" class="Slide (strict)"("Visible"=FALSE) -> ()  [unwired: 2 in, 2 out]
              }
              frame "White Balance  **" {
                n131 = Index Array(array=w216, index=1) -> (element=w217:cluster{string[]})
                n132 = call <vilib>:"NT Read String.vi"("Name"=w219) -> ("String"=w218:string)  [unwired: 9 in, 1 out]
                n133 = Unbundle(w217) -> (w214:string[])
                n134 = Match First String(2:w214, 3:w218) -> (0:w213:i32)  [unwired: 1 out]
                n135 = property on="Test Ring" class="Ring (strict)"("Value"=w213, "Strings []"=w214) -> ()  [unwired: 2 in, 2 out]
                n136 = property on="Test Ring" class="Ring (strict)"("Visible"=TRUE) -> ()  [unwired: 2 in, 2 out]
                n137 = property on="Test Slider" class="Slide (strict)"("Visible"=FALSE) -> ()  [unwired: 2 in, 2 out]
              }
              frame "Exposure  **" {
                n138 = Index Array(array=w225, index=2) -> (element=w226:cluster{string[]})
                n139 = call <vilib>:"NT Read String.vi"("Name"=w228) -> ("String"=w227:string)  [unwired: 9 in, 1 out]
                n140 = Unbundle(w226) -> (w222:string[])
                n141 = Match First String(2:w222, 3:w227) -> (0:w223:i32)  [unwired: 1 out]
                n142 = property on="Test Ring" class="Ring (strict)"("Value"=w223, "Strings []"=w222) -> ()  [unwired: 2 in, 2 out]
                n143 = property on="Test Ring" class="Ring (strict)"("Visible"=TRUE) -> ()  [unwired: 2 in, 2 out]
                n144 = property on="Test Slider" class="Slide (strict)"("Visible"=FALSE) -> ()  [unwired: 2 in, 2 out]
              }
              frame "Exposure Priority  **" {
                n145 = Index Array(array=w234, index=3) -> (element=w235:cluster{string[]})
                n146 = call <vilib>:"NT Read String.vi"("Name"=w237) -> ("String"=w236:string)  [unwired: 9 in, 1 out]
                n147 = Unbundle(w235) -> (w231:string[])
                n148 = Match First String(2:w231, 3:w236) -> (0:w232:i32)  [unwired: 1 out]
                n149 = property on="Test Ring" class="Ring (strict)"("Value"=w232, "Strings []"=w231) -> ()  [unwired: 2 in, 2 out]
                n150 = property on="Test Ring" class="Ring (strict)"("Visible"=TRUE) -> ()  [unwired: 2 in, 2 out]
                n151 = property on="Test Slider" class="Slide (strict)"("Visible"=FALSE) -> ()  [unwired: 2 in, 2 out]
              }
              frame "Color Enable  **" {
                n152 = Index Array(array=w243, index=4) -> (element=w244:cluster{string[]})
                n153 = call <vilib>:"NT Read String.vi"("Name"=w246) -> ("String"=w245:string)  [unwired: 9 in, 1 out]
                n154 = Unbundle(w244) -> (w240:string[])
                n155 = Match First String(2:w240, 3:w245) -> (0:w241:i32)  [unwired: 1 out]
                n156 = property on="Test Ring" class="Ring (strict)"("Value"=w241, "Strings []"=w240) -> ()  [unwired: 2 in, 2 out]
                n157 = property on="Test Ring" class="Ring (strict)"("Visible"=TRUE) -> ()  [unwired: 2 in, 2 out]
                n158 = property on="Test Slider" class="Slide (strict)"("Visible"=FALSE) -> ()  [unwired: 2 in, 2 out]
              }
              frame Default {
                n159 = property on="Test Ring" class="Ring (strict)"("Visible"=FALSE) -> ()  [unwired: 2 in, 2 out]
                n160 = property on="Test Slider" class="Slide (strict)"("Visible"=FALSE) -> ()  [unwired: 2 in, 2 out]
              }
              frame "Brightness  **", "Color Level  **", "Compression  **", "FPS  **", "Sharpness  **" {
                n161 = call <vilib>:"NT Read Number.vi"("Name"=w252) -> ("Numeric"=w251:dbl)  [unwired: 9 in, 1 out]
                n162 = local write "Test Slider"(w251) -> ()
                n163 = property on="Test Slider" class="Slide (strict)"("Visible"=TRUE, "Scale.Maximum"=100.0 ("Scale.Range:Maximum")) -> ()  [unwired: 2 in, 2 out]
                n164 = property on="Test Ring" class="Ring (strict)"("Visible"=FALSE) -> ()  [unwired: 2 in, 2 out]
              }
            }
          }
        }
        n165 = property on="Progress" class="Clust (strict)"("Visible"=FALSE) -> ()  [unwired: 2 in, 2 out]
      }
      event "Test Name": Mouse Enter {
        # "Populate the ring with the list of tests"
        n166 = event-data() -> ()  [unwired: 1 in, 1 out]
        n167 = call <vilib>:"NT Read String Array.vi"("Name"="TestMode/TestList") -> ("String Array"=w260:string[])  [unwired: 9 in, 1 out]
        n168 = Build Array (concatenate)("Select the test to run...", w260) -> (w259:string[])
        n169 = property on="Test Name" class="Ring (strict)"("Strings []"=w259) -> ()  [unwired: 2 in, 2 out]
      }
      event "Test Name": Value Change {
        w262 = FALSE ("Visible")
        # "Tell the robot the test name to run"
        n170 = event-data() -> ("NewVal"=w266:u16)  [unwired: 1 in]
        n171 = property on="Test Name" class="Ring (strict)"() -> ("Strings []"=w267:string[])  [unwired: 2 in, 2 out]
        n172 = local write "Progress"(T4 {"Test Progress"=0, "Test Progress Text"=""} ("Progress")) -> ()
        n173 = Index Array(array=w267, index=w266) -> (element=w265:string)
        n174 = call <vilib>:"NT Write String.vi"("String"=w265, "Name"="TestMode/TestName") -> ()  [unwired: 9 in, 1 out]
        n175 = property on="Progress" class="Clust (strict)"("Visible"=TRUE) -> ()  [unwired: 2 in, 2 out]
        n176 = property on="Motor" class="Clust (strict)"("Visible"=w262) -> ()  [unwired: 2 in, 2 out]
        n177 = property on="Test Slider" class="Slide (strict)"("Visible"=w262) -> ()  [unwired: 2 in, 2 out]
        n178 = property on="On/Off" class="Bool (strict)"("Visible"=w262) -> ()  [unwired: 2 in, 2 out]
        n179 = property on="Rev/Fwd" class="Clust (strict)"("Visible"=w262) -> ()  [unwired: 2 in, 2 out]
        n180 = property on="Test Ring" class="Ring (strict)"("Visible"=w262) -> ()  [unwired: 2 in, 2 out]
      }
      event "Listbox": Double Click {
        # "Shift clears all"
        # "Update symbols on the listbox"
        n181 = event-data() -> ("PlatMods.Shift"=w270:bool, "Row"=w272:i32)  [unwired: 1 in]
        n182 = case shown="True" w270 {
          tunnel: w272 -> [w276 _]
          tunnel: 1 -> [w275 _]
          frame False {
            n183 = property on="Listbox" class="LstBox (strict)"() -> ("Item Symbols"=w274:i32[])  [unwired: 2 in, 2 out]
            n184 = Replace Array Subset(array=w274, new element=w275, index=w276) -> (w273:i32[])
            n185 = property on="Listbox" class="LstBox (strict)"("Item Symbols"=w273) -> ()  [unwired: 2 in, 2 out]
          }
          frame True {
            w277 = 0 ("Top Row")
            n186 = property on="Listbox" class="LstBox (strict)"() -> ("Number of Rows"=w279:u32)  [unwired: 2 in, 2 out]
            n187 = Initialize Array(0, w279) -> (w278:i32[])
            n188 = property on="Listbox" class="LstBox (strict)"("Top Row"=w277, "Value"=w277, "Item Symbols"=w278) -> ()  [unwired: 2 in, 2 out]
          }
        }
      }
      event "Listbox": Key Down {
        # "Update symbols on the listbox\nLeft and right keys check and uncheck"
        n189 = event-data() -> ("VKey"=w283:T16)  [unwired: 1 in]
        n190 = case shown="\"Left\", \"Right\"" w283 {
          selector: w283 -> [w288 _]
          tunnel: eventvkey."Left" ("VKey") -> [w286 _]
          frame "Left", "Right" {
            n191 = Equal?(x=w286, y=w288) -> (x = y?=w287:bool)
            n192 = Select(t=0, s=w287, f=1) -> (s? t:f=w289:i32)
            n193 = property on="Listbox" class="LstBox (strict)"() -> ("Item Symbols"=w292:i32[])  [unwired: 2 in, 2 out]
            n194 = Replace Array Subset(array=w292, new element=w289, index="Listbox") -> (w291:i32[])
            n195 = property on="Listbox" class="LstBox (strict)"("Item Symbols"=w291) -> ()  [unwired: 2 in, 2 out]
          }
          frame Default {
          }
        }
      }
      event "DB Camera Config": Value Change {
        # "Show or hide the cluster of controls, store in ini file"
        n196 = event-data() -> ("NewVal"=w296:bool)  [unwired: 1 in]
        n197 = case shown="False" w296 {
          tunnel: w295 -> [w305 _]
          tunnel: [w298 w316] -> w294
          tunnel: w293 -> [w297 w316]
          frame False {
            w312 = "Camera"
            w315 = FALSE ("Visible")
            n198 = local read "Camera Settings Old"() -> (w304:T2)
            n199 = Index Array(array=w305) -> (element=w308:cluster{string[]})  [unwired: 1 in]
            n200 = Unbundle(w304) -> ("Frame Rate"=w303:i32, "Compression"=w302:i32, "Size"=w306:u16)  [unwired: 1 out]
            n201 = Unbundle(w308) -> (w307:string[])
            n202 = Index Array(array=w307, index=w306) -> (element=w301:string)
            n203 = call-poly <vilib>:"Write Key.vi"("section"=w312, "value"=w301, "key"="Size", "refnum"=w297) -> ("refnum out"=w314:T14)  [unwired: 2 in, 5 out]
            n204 = call-poly <vilib>:"Write Key.vi"("section"=w312, "value"=w303, "key"="FrameRate", "refnum"=w314) -> ("refnum out"=w313:T14)  [unwired: 1 in, 6 out]
            n205 = property on="Camera Settings Old" class="Clust (strict)"("Visible"=w315) -> ()  [unwired: 2 in, 2 out]
            n206 = local write "DB Camera Config"(w315) -> ()
            n207 = call-poly <vilib>:"Write Key.vi"("section"=w312, "value"=w302, "key"="Compression", "refnum"=w313) -> ("refnum out"=w299:T14)  [unwired: 1 in, 6 out]
            n208 = call <vilib>:"Close Config Data.vi"("refnum"=w299) -> ("file path"=w300:path)  [unwired: 2 in, 8 out]
            n209 = call <vilib>:"Open Config Data.vi"("configuration file path"=w300) -> ("refnum"=w298:T14)  [unwired: 8 in, 2 out]
          }
          frame True {
            n210 = property on="Camera Settings Old" class="Clust (strict)"("Visible"=TRUE) -> ()  [unwired: 2 in, 2 out]
          }
        }
      }
      event "Camera Settings Old": Value Change {
        # "Update summary string when any elements of DB camera change"
        n211 = event-data() -> ("NewVal"=w329:T2)  [unwired: 1 in]
        n212 = Index Array(array=w325) -> (element=w324:cluster{string[]})  [unwired: 1 in]
        n213 = Unbundle(w329) -> ("Frame Rate"=w320:i32, "Compression"=w319:i32, "Size"=w322:u16)  [unwired: 1 out]
        n214 = Unbundle(w324) -> (w323:string[])
        n215 = Index Array(array=w323, index=w322) -> (element=w321:string)
        n216 = Format Into String(format string="%s   %dfps   %d%%", w321, w320, w319) -> (resulting string=w326:string)  [unwired: 2 in, 1 out]
        n217 = Build Array(w326) -> (w327:string[])
        n218 = property on="DB Camera Config" class="Bool (strict)"("Strings [4]"=w327) -> ()  [unwired: 2 in, 2 out]
      }
      event "Motor.Enable": Value Change {
        # "When the test mode otor enable helper is set, update that\ntree row item's value"
        n219 = event-data() -> ("NewVal"=w335:bool)  [unwired: 1 in]
        n220 = Unbundle("Motor") -> ("Value"=w334:dbl)  [unwired: 1 out]
        n221 = Select(t=w334, s=w335, f=0.0) -> (s? t:f=w332:dbl)
        n222 = call <vilib>:"NT Write Number.vi"("Numeric"=w332, "Name"=w331) -> ()  [unwired: 9 in, 1 out]
      }
      event "Test Slider": Value Change {
        # "When the test mode slider helper is set, update that\ntree row item's value"
        n223 = event-data() -> ("NewVal"=w338:dbl)  [unwired: 1 in]
        n224 = call <vilib>:"NT Write Number.vi"("Numeric"=w338, "Name"=w339) -> ()  [unwired: 9 in, 1 out]
      }
      event "On/Off": Value Change {
        # "When the test mode on/off helper value is set, update that\ntree row item's value"
        n225 = event-data() -> ("NewVal"=w343:bool)  [unwired: 1 in]
        n226 = Boolean To (0,1)(Boolean=w343) -> (0, 1=w342:i16)
        n227 = call <vilib>:"NT Write Number.vi"("Numeric"=w342, "Name"=w341) -> ()  [unwired: 9 in, 1 out]
      }
      event "Rev/Fwd": Value Change {
        # "When the test mode helper value for relays is set, update that\ntree row item's value"
        n228 = event-data() -> ("NewVal.Forward"=w351:bool, "NewVal.Reverse"=w350:bool)  [unwired: 1 in]
        n229 = Boolean To (0,1)(Boolean=w351) -> (0, 1=w347:i16)
        n230 = Boolean To (0,1)(Boolean=w350) -> (0, 1=w349:i16)
        n231 = Negate(x=w349) -> (-x=w348:i16)
        n232 = Add(x=w347, y=w348) -> (x+y=w346:i16)
        n233 = call <vilib>:"NT Write Number.vi"("Numeric"=w346, "Name"=w345) -> ()  [unwired: 9 in, 1 out]
      }
      event "Test Ring": Value Change {
        # "When a test mode helper value is selected from the ring,\nset the tree item's variable to the string value"
        n234 = event-data() -> ("NewVal"=w355:u16)  [unwired: 1 in]
        n235 = property on="Test Ring" class="Ring (strict)"() -> ("Strings []"=w356:string[])  [unwired: 2 in, 2 out]
        n236 = Index Array(array=w356, index=w355) -> (element=w354:string)
        n237 = call <vilib>:"NT Write String.vi"("String"=w354, "Name"=w353) -> ()  [unwired: 9 in, 1 out]
      }
      event "Rec Mode": Value Change {
        # "Update globals for recording mode and path to read log from.\nClear when logging and let NetworkTables set path for vision to\nuse."
        n238 = event-data() -> ("NewVal"=w366:enum32{"Stop", "Record", "Playback"})  [unwired: 1 in]
        n239 = global write "WPI_DashboardLogging Global.vi" "Logging Filename"(path "") -> ()
        n240 = case shown="\"Playback\"" w366 {
          tunnel: w365 -> [_ w368 w376]
          tunnel: [_ _ w375] -> w362
          tunnel: [_ _ w374] -> _
          tunnel: w360 -> [_ _ w372]
          tunnel: cluster{i32, i32} {-250, 170} -> [_ _ w371]
          tunnel: [_ _ T17 {"Image Size"=TRUE, "Image Type"=TRUE, "Pixel Value"=TRUE, "ROI Information"=TRUE, "Zoom Factor"=FALSE} ("Image Information Shown:All Elements")] -> w358
          tunnel: [_ _ TRUE ("Zoom Factor")] -> w357
          frame Default {
          }
          frame "Stop", "Record" {
            # "Place Window too"
            n241 = invoke class="VI" method="FP.Close"(reference=w368) -> (reference out=w367:refnum<vi>)  [unwired: 2 in, 2 out]
            n242 = invoke class="VI" method="Abort VI"(reference=w367) -> ()  [unwired: 2 in, 3 out]
          }
          frame "Playback" {
            n243 = call "Open Playback Panel.vi"("Offset"=w371, "DB VI Ref"=w372, "Playback in"=w376) -> ("Playback out"=w373:refnum<vi>)  [unwired: 8 in]
            n244 = register-events(w373) -> (reference out=w375:refnum<event-registration>, error out=w374:errorcluster)  [unwired: 2 in]
          }
        }
        n245 = global write "WPI_DashboardLogging Global.vi" "Recording"(w366) -> ()
        n246 = property on="Camera Image" class="ImageControl"("Image Information Shown"=w358, "Image Information Visible"=w357) -> ()  [unwired: 2 in, 2 out]
        n247 = call <vilib>:"WPI_DashboardNT Log FieldName Cache.vi"("Operation"=enum16{"Lookup/Add", "Index", "Clear"}."Clear") -> ()  [unwired: 8 in, 3 out]
      }
      event Panel Close {
        w377 = enum32{"Stop", "Record", "Playback"}."Stop" ("Rec Mode")
        # "Playback window has been closed, abort"
        n248 = event-data() -> ()  [unwired: 1 in, 4 out]
        n249 = local write "Rec Mode"(w377) -> ()
        n250 = global write "WPI_DashboardLogging Global.vi" "Recording"(w377) -> ()
      }
      event Panel Close {
        # "Abort playback window and ourself"
        n251 = event-data() -> ()  [unwired: 1 in, 4 out]
        n252 = invoke class="VI" method="FP.Close"(reference=w382) -> (reference out=w381:refnum<vi>)  [unwired: 2 in, 2 out]
        n253 = invoke class="VI" method="Abort VI"(reference=w381) -> (error out=w380:errorcluster)  [unwired: 2 in, 2 out]
        n254 = invoke class="VI" method="Abort VI"(error in=w380) -> ()  [unwired: 2 in, 3 out]
      }
      event "Vision": Value Change {
        # "Enable/Disable Compression slider.\nHW USB is hard-coded into the camera"
        n255 = event-data() -> ("NewVal"=w388:u16)  [unwired: 1 in]
        n256 = Equal?(x=w388, y=u32 2 ("milliseconds to wait")) -> (x = y?=w386:bool)
        n257 = Select(t=T18."Disabled and Grayed Out" ("Disabled"), s=w386, f=T18."Enabled" ("Disabled")) -> (s? t:f=w383:T18)
        n258 = property on="Compression" class="Slide (strict)"("DisabledEnum"=w383) -> ()  [unwired: 2 in, 2 out]
      }
    }
  }
  n259 = while {
    tunnel: w38 -> [w391]
    i -> [w394]
    stop <- FALSE stop-if-true
    n260 = Wait (ms)(milliseconds to wait=u32 100) -> ()  [unwired: 1 out]
    n261 = case shown="\"Playback\"" "Rec Mode" {
      tunnel: w394 -> [_ _ w409]
      tunnel: [u32 2829099 ("Base Color") u32 11141120 ("Target Color") w398] -> w390
      frame "Stop", Default {
        # "Reset the color, extra updates don't cost much"
      }
      frame "Record" {
      }
      frame "Playback" {
        # "Playback"
        n262 = Quotient & Remainder(x=w409, y=u32 50 ("milliseconds to wait")) -> (x-y*floor(x/y)=w405:u32)  [unwired: 1 out]
        n263 = Divide(x=w405, y=u32 50 ("milliseconds to wait")) -> (x/y=w402:dbl)
        n264 = Multiply(x=6.283185307179586, y=w402) -> (x*y=w407:dbl)
        n265 = Sine(x=w407) -> (sin(x)=w406:dbl)
        n266 = Absolute Value(x=w406) -> (abs(x)=w399:dbl)
        n267 = call "Interpolate RGB Color.vi"("Proportion"=w399, "Target Color"=u32 30976, "Base Color"=u32 2829099) -> ("Result Color"=w398:u32)  [unwired: 8 in]
      }
    }
    n268 = property class="Pane"(reference=w391, "PaneColor"=w390) -> ()  [unwired: 1 in, 2 out]
  }
  n269 = TCP Create Listener(10:u16 1741 ("timeout ms (25000)")) -> (3:w1:refnum<k5>)  [unwired: 4 in, 2 out]
  n270 = while {
    tunnel: w1 -> [w411]
    stop <- FALSE stop-if-true
    n271 = TCP Wait On Listener(11:w411) -> (4:w410:refnum<k5>)  [unwired: 3 in, 4 out]
    n272 = local write "TCP"(w410) -> ()
  }
  n273 = property on="On/Off" class="Bool (strict)"("Visible"=w6) -> ()  [unwired: 2 in, 2 out]
  n274 = property on="Motor" class="Clust (strict)"("Visible"=w6) -> ()  [unwired: 2 in, 2 out]
  n275 = property on="Progress" class="Clust (strict)"("Visible"=w6) -> ()  [unwired: 2 in, 2 out]
  n276 = property on="Test Ring" class="Ring (strict)"("Visible"=w6) -> ()  [unwired: 2 in, 2 out]
  n277 = property on="Rev/Fwd" class="Clust (strict)"("Visible"=w6) -> ()  [unwired: 2 in, 2 out]
  n278 = property on="Camera Settings Old" class="Clust (strict)"("Visible"=w6) -> ()  [unwired: 2 in, 2 out]
  n279 = local write "DB Camera Config"(w6) -> ()
  n280 = global write "WPI_DashboardLogging Global.vi" "Recording"(w32) -> ()
  n281 = local write "Rec Mode"(w32) -> ()
